vi "4.1.1.-SubVI Histograma.vi"(11 "imagen":T1) -> (1 "G":i32, 2 "R":i32, 3 "Histograma":cluster{"Array":i32[], dbl[]}[](array[cluster]), 4 "B":i32)   [LabVIEW 2020]
uses:
  <vilib>/picture/picture.llb/imagedata.ctl
  2fa15919-2e5a-46f2-a123-77936c30e24e.vi
  bfc831ed-f1e7-4cb6-be6f-2d9d4744283d.vi
  995d4483-f2fe-408d-a5a8-8c89eedf084d.vi
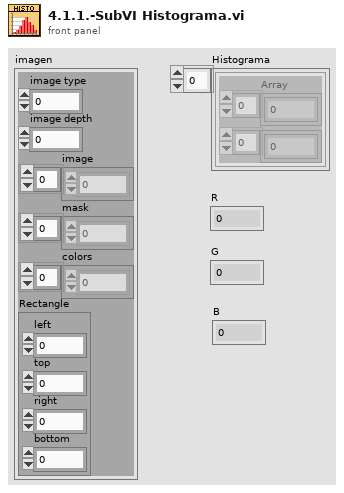
[diagram p1: front panel]
types:
  T1 = typedef "imagedata.ctl" = cluster{"image type":i32, "image depth":i32, "image":u8[], "mask":u8[], "colors":u32[], "Rectangle":cluster{"left":i16, "top":i16, "right":i16, "bottom":i16}}
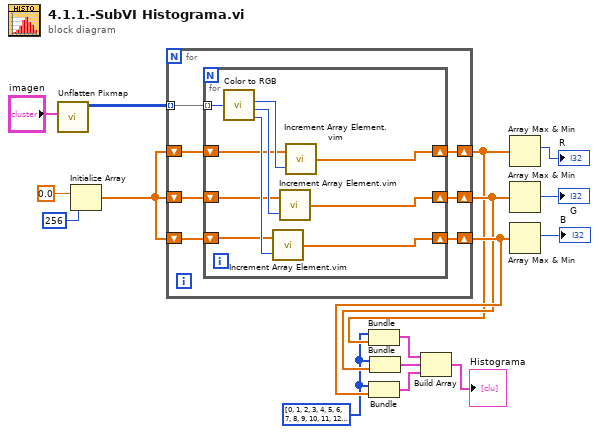
[diagram p0: block diagram]
diagram:
  w7 = i32[] [0, 1, 2, 3, 4, 5, 6, 7, 8, 9, 10, 11, 12, 13, 14, 15, 16, 17, 18, 19, 20, 21, 22, 23, 24, 25, 26, 27, 28, 29, 30, 31, 32, 33, 34, 35, 36, 37, 38, 39, 40, 41, 42, 43, 44, 45, 46, 47, 48, 49, 50, 51, 52, 53, 54, 55, 56, 57, 58, 59, 60, 61, 62, 63, 64, 65, 66, 67, 68, 69, 70, 71, 72, 73, 74, 75, 76, 77, 78, 79, 80, 81, 82, 83, 84, 85, 86, 87, 88, 89, 90, 91, 92, 93, 94, 95, 96, 97, 98, 99, 100, 101, 102, 103, 104, 105, 106, 107, 108, 109, 110, 111, 112, 113, 114, 115, 116, 117, 118, 119, 120, 121, 122, 123, 124, 125, 126, 127, 128, 129, 130, 131, 132, 133, 134, 135, 136, 137, 138, 139, 140, 141, 142, 143, 144, 145, 146, 147, 148, 149, 150, 151, 152, 153, 154, 155, 156, 157, 158, 159, 160, 161, 162, 163, 164, 165, 166, 167, 168, 169, 170, 171, 172, 173, 174, 175, 176, 177, 178, 179, 180, 181, 182, 183, 184, 185, 186, 187, 188, 189, 190, 191, 192, 193, 194, 195, 196, 197, 198, 199, 200, 201, 202, 203, 204, 205, 206, 207, 208, 209, 210, 211, 212, 213, 214, 215, 216, 217, 218, 219, 220, 221, 222, 223, 224, 225, 226, 227, 228, 229, 230, 231, 232, 233, 234, 235, 236, 237, 238, 239, 240, 241, 242, 243, 244, 245, 246, 247, 248, 249, 250, 251, 252, 253, 254, 255] ("Array")
  n1 = call <vilib>:"Unflatten Pixmap.vi"("image data"="imagen") -> ("24-bit pixmap"=w3:u32[][])  [unwired: 4 in, 6 out]
  n2 = Initialize Array "Initialize Array"(0.0 ("element"), 256 ("dimension size")) -> (w1:dbl[])
  n3 = for {
    tunnel: w3 -> [w23] mode=indexing
    shift-right: [w22] -> w8
    shift-left: w1 -> [w21]
    shift-right: [w20] -> w9
    shift-left: w1 -> [w19]
    shift-right: [w18] -> w10
    shift-left: w1 -> [w17]
    n4 = for {
      tunnel: w23 -> [w33] mode=indexing
      shift-right: [w24] -> w22
      shift-left: w21 -> [w25]
      shift-right: [w29] -> w20
      shift-left: w19 -> [w26]
      shift-right: [w28] -> w18
      shift-left: w17 -> [w27]
      n5 = call <vilib>:"Color to RGB.vi"("Color"=w33) -> ("R"=w32:u8, "G"=w30:u8, "B"=w31:u8)  [unwired: 1 out]
      n6 = call "Increment Array Element.vim"("index"=w31, "array in"=w27) -> ("array out"=w28:dbl[])
      n7 = call "Increment Array Element.vim"("index"=w30, "array in"=w26) -> ("array out"=w29:dbl[])
      n8 = call "Increment Array Element.vim"("index"=w32, "array in"=w25) -> ("array out"=w24:dbl[])
    }
  }
  n9 = Bundle("Array"=w7, w8) -> (w6:cluster{"Array":i32[], dbl[]})  [unwired: 1 in]
  n10 = Bundle("Array"=w7, w10) -> (w4:cluster{"Array":i32[], dbl[]})  [unwired: 1 in]
  n11 = Bundle("Array"=w7, w9) -> (w5:cluster{"Array":i32[], dbl[]})  [unwired: 1 in]
  n12 = Build Array "Build Array"(w6, w5, w4) -> (→"Histograma":cluster{"Array":i32[], dbl[]}[])
  n13 = Array Max & Min(array=w8) -> (max index (indices)=→"R":i32)  [unwired: 3 out]
  n14 = Array Max & Min(array=w9) -> (max index (indices)=→"G":i32)  [unwired: 3 out]
  n15 = Array Max & Min(array=w10) -> (max index (indices)=→"B":i32)  [unwired: 3 out]
